vi "Three Button Dialog CORE.vi"(4 "Allow user to close window? (TRUE)":bool=TRUE, 5 "Justify Message (Left)":enum16{"Left", "Center", "Right"}(ring), 6 "Keyboard Shortcuts (Left is <Enter>)":T1={"Left Button Key Shortcut"={"Control"=FALSE, "Shift"=FALSE, "Key"="<Enter>"}, "Center Button Key Shortcut"={"Control"=FALSE, "Shift"=FALSE, "Key"=""}, "Right Button Key Shortcut"={"Control"=FALSE, "Shift"=FALSE, "Key"=""}}, 7 "Window Title (\"\")":string, 8 "Right Button Text (\"Cancel\")":string="Cancel", 9 "Center Button Text (\"No\")":string="No", 10 "Left Button Text (\"Yes\")":string="Yes", 11 "message":string) -> (3 "Which Button?":T2(ring)=enum."Center Button")   [LabVIEW 2020]
doc: "Displays text in a dialog with three buttons. The output enum indicates which of the three buttons the user chose, or it indicates that the user closed the dialog without making any choice."
panel:
  in  "OK":string="OK"
  out "C-Message":string
  in  "Right Button":bool
  in  "Center Button":bool
  in  "Left Button":bool
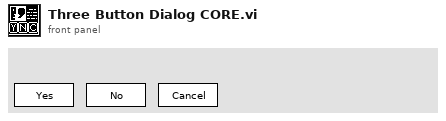
[diagram p1: front panel]
types:
  T1 = cluster{"Left Button Key Shortcut":cluster{"Control":bool, "Shift":bool, "Key":string}, "Center Button Key Shortcut":cluster{"Control":bool, "Shift":bool, "Key":string}, "Right Button Key Shortcut":cluster{"Control":bool, "Shift":bool, "Key":string}}
  T2 = enum16{"Left Button", "Center Button", "Right Button", "Window Close"}
  T3 = cluster{"left":i16, "top":i16, "right":i16, "bottom":i16}
  T4 = cluster{"Control":bool, "Shift":bool, "Key":string}
  T5 = cluster{bool, "Control":bool, "Shift":bool, "Key":string}
  T6 = cluster{"Left":i16, "Top":i16, "Right":i16, "Bottom":i16}
  T7 = typedef "LVRectTypeDef.ctl" = cluster{"Left":i16, "Top":i16, "Right":i16, "Bottom":i16}
  T8 = typedef "LVPointTypeDef.ctl" = cluster{"Horizontal":i16, "Vertical":i16}
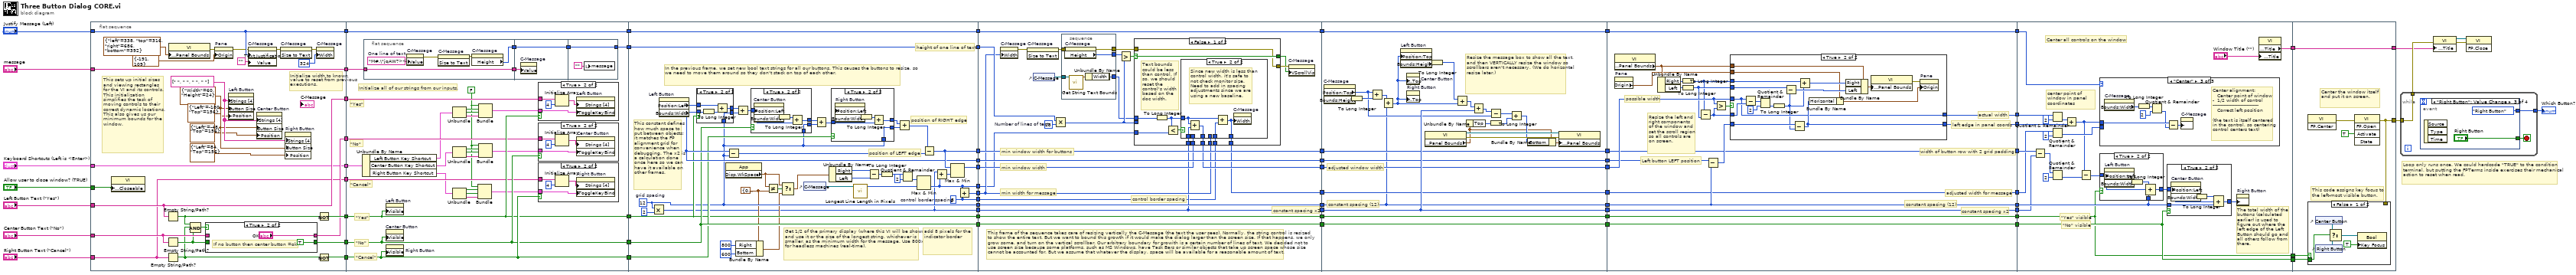
[diagram p0: block diagram]
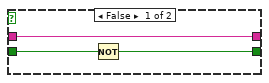
[diagram p2: hidden frame]
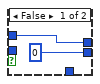
[diagram p6: hidden frame]
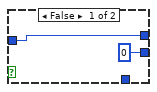
[diagram p7: hidden frame]
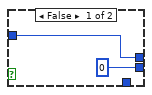
[diagram p8: hidden frame]
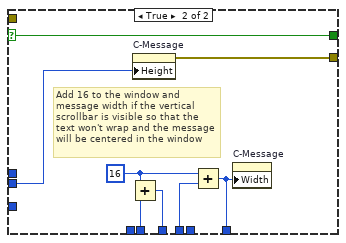
[diagram p10: hidden frame]
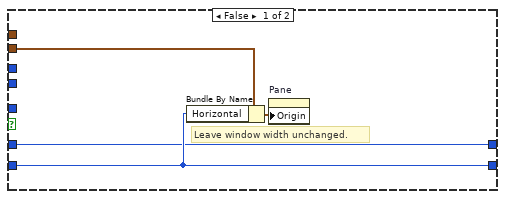
[diagram p11: hidden frame]
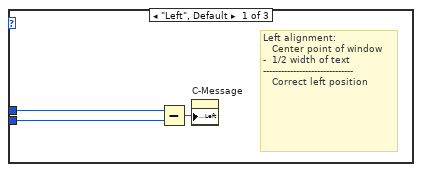
[diagram p12: hidden frame]
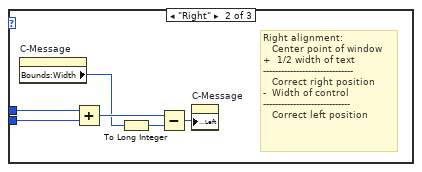
[diagram p13: hidden frame]
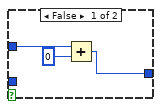
[diagram p14: hidden frame]
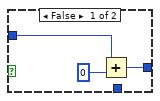
[diagram p15: hidden frame]
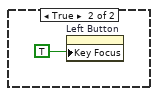
[diagram p16: hidden frame]
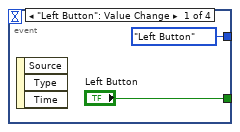
[diagram p17: hidden frame]
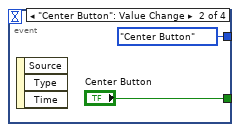
[diagram p18: hidden frame]
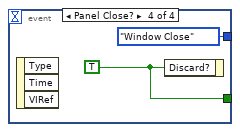
[diagram p19: hidden frame]
diagram:
  # "Loop only runs once. We could hardcode \"TRUE\" to the condition terminal, but putting the FPTerms inside exercises their mechanical action to reset when read."
  n1 = flat-sequence {
    tunnel: [w87] -> w15
    tunnel: [w89] -> w14
    tunnel: [w88] -> w13
    tunnel: [w83] -> w12
    tunnel: [w84] -> w11
    tunnel: [w81] -> w10
    tunnel: [w80] -> w9
    tunnel: "Left Button Text (\"Yes\")" -> [w83]
    tunnel: "Center Button Text (\"No\")" -> [w82]
    tunnel: "Right Button Text (\"Cancel\")" -> [w81]
    tunnel: "Justify Message (Left)" -> [w80]
    tunnel: "Keyboard Shortcuts (Left is <Enter>)" -> [w77]
    tunnel: [w77] -> w8
    tunnel: "message" -> [w76]
    tunnel: [w76] -> w7
    tunnel: "Allow user to close window? (TRUE)" -> [w75]
    tunnel: w15 -> [w131]
    tunnel: [w131] -> w65
    tunnel: w14 -> [w130]
    tunnel: [w130] -> w64
    tunnel: w13 -> [w129]
    tunnel: [w129] -> w63
    tunnel: w12 -> [w128]
    tunnel: w11 -> [w127]
    tunnel: w10 -> [w126]
    tunnel: w9 -> [w125]
    tunnel: [w125] -> w62
    tunnel: [w121] -> w61
    tunnel: w8 -> [w124]
    tunnel: w7 -> [w120]
    tunnel: [w192] -> w60
    tunnel: [w189] -> w59
    tunnel: [w188] -> w58
    tunnel: [w171] -> w57
    tunnel: [w153] -> w56
    tunnel: w65 -> [w181]
    tunnel: w64 -> [w183]
    tunnel: [w183] -> w55
    tunnel: w63 -> [w179]
    tunnel: [w179] -> w54
    tunnel: [w164] -> w53
    tunnel: w62 -> [w174]
    tunnel: [w174] -> w52
    tunnel: w61 -> [w173]
    tunnel: [w173] -> w51
    tunnel: [w162] -> w4
    tunnel: [w161] -> w3
    tunnel: w60 -> [w227]
    tunnel: [w226] -> w50
    tunnel: w59 -> [w233]
    tunnel: [w233] -> w49
    tunnel: w58 -> [w232]
    tunnel: [w232] -> w48
    tunnel: w57 -> [w231]
    tunnel: [w231] -> w47
    tunnel: w56 -> [w220]
    tunnel: [w220] -> w46
    tunnel: w55 -> [w230]
    tunnel: [w230] -> w45
    tunnel: w54 -> [w229]
    tunnel: [w229] -> w44
    tunnel: w53 -> [w221]
    tunnel: [w225] -> w43
    tunnel: w52 -> [w228]
    tunnel: [w228] -> w42
    tunnel: w51 -> [w223]
    tunnel: w4 -> [w219]
    tunnel: w3 -> [w218]
    tunnel: w50 -> [w282]
    tunnel: [w282] -> w41
    tunnel: w49 -> [w281]
    tunnel: [w281] -> w40
    tunnel: w48 -> [w280]
    tunnel: [w280] -> w39
    tunnel: w47 -> [w273]
    tunnel: [w273] -> w38
    tunnel: w46 -> [w290]
    tunnel: [w290] -> w37
    tunnel: w45 -> [w279]
    tunnel: [w279] -> w36
    tunnel: w44 -> [w278]
    tunnel: [w278] -> w35
    tunnel: w43 -> [w277]
    tunnel: [w277] -> w34
    tunnel: w42 -> [w276]
    tunnel: [w276] -> w33
    tunnel: w41 -> [w317]
    tunnel: [w312] -> w32
    tunnel: w40 -> [w305]
    tunnel: [w305] -> w31
    tunnel: w39 -> [w311]
    tunnel: w38 -> [w310]
    tunnel: [w310] -> w30
    tunnel: w37 -> [w304]
    tunnel: [w304] -> w29
    tunnel: [w308] -> w28
    tunnel: w36 -> [w303]
    tunnel: [w303] -> w27
    tunnel: w35 -> [w302]
    tunnel: [w302] -> w26
    tunnel: w34 -> [w299]
    tunnel: [w299] -> w25
    tunnel: w33 -> [w301]
    tunnel: [w301] -> w24
    tunnel: [w342] -> w23
    tunnel: w32 -> [w361]
    tunnel: w31 -> [w354]
    tunnel: w30 -> [w358]
    tunnel: w29 -> [w353]
    tunnel: w28 -> [w360]
    tunnel: w27 -> [w341]
    tunnel: w26 -> [w340]
    tunnel: w25 -> [w346]
    tunnel: w24 -> [w347]
    tunnel: [w341] -> w6
    tunnel: [w340] -> w5
    tunnel: [w396] -> w68
    tunnel: [w398] -> w66
    tunnel: w23 -> [w398]
    tunnel: w6 -> [w394]
    tunnel: w5 -> [w395]
    frame #0 {
      w97 = string[] [" ", " ", " ", " "] ("Strings [4]")
      w96 = cluster{"Width":u32, "Height":u32} {"Width"=60, "Height"=24} ("Button Size")
      # "Initialize width to known value to reset from previous executions."
      # "This sets up initial sizes and viewing rectangles\nfor the VI and its controls. This initialization\nsimplifies the task of moving controls to their\ncorrect dynamic locations. This also gives us our\nminimum bounds for the window."
      n2 = property class="VI"("Front Panel Window:Closeable"=w75) -> ()  [unwired: 2 in, 2 out]
      n3 = Empty String/Path?(string/path=w83) -> (empty?=w91:bool)
      n4 = Empty String/Path?(string/path=w82) -> (empty?=w79:bool)
      n5 = Empty String/Path?(string/path=w81) -> (empty?=w78:bool)
      n6 = property class="VI"("Front Panel Window:Panel Bounds"=T3 {"left"=338, "top"=316, "right"=686, "bottom"=392} ("Front Panel.PanelBounds")) -> (error out=w74:errorcluster)  [unwired: 2 in, 1 out]
      n7 = Compound Arithmetic op=AND(w91, w78, w79) -> (w90:bool)
      n8 = case shown="True" w90 {
        tunnel: w79 -> [w100 _]
        tunnel: [w99 TRUE] -> w89
        tunnel: w82 -> [w98 _]
        tunnel: [w98 "OK"] -> w84
        frame False {
          n9 = Not(x=w100) -> (.not. x?=w99:bool)
        }
        frame True {
          # "If no button then center button =ok"
        }
      }
      n10 = property on="Pane" class="Pane"(error in=w74, "Origin"=cluster{"Horizontal":i16, "Vertical":i16} {"Horizontal"=-191, "Vertical"=109} ("Front Panel.Origin")) -> (error out=w73:errorcluster)  [unwired: 1 in, 1 out]
      n11 = property on="Left Button" class="Bool"("Strings [4]"=w97, "Button Size"=w96, "Position"=cluster{"Left":i32, "Top":i32} {"Left"=-180, "Top"=156}) -> ()  [unwired: 2 in, 2 out]
      n12 = property on="C-Message" class="Str"(error in=w73, "Text.Justification"=w80, "Value"="") -> (error out=w92:errorcluster)  [unwired: 1 in, 1 out]
      n13 = property on="Center Button" class="Bool"("Strings [4]"=w97, "Button Size"=w96, "Position"=cluster{"Left":i32, "Top":i32} {"Left"=-48, "Top"=156}) -> ()  [unwired: 2 in, 2 out]
      n14 = invoke on="C-Message" class="Str" method="Size to Text"(error in=w92) -> (error out=w71:errorcluster)  [unwired: 2 in, 2 out]
      n15 = property on="Right Button" class="Bool"("Strings [4]"=w97, "Button Size"=w96, "Position"=cluster{"Left":i32, "Top":i32} {"Left"=84, "Top"=156}) -> ()  [unwired: 2 in, 2 out]
      n16 = property on="C-Message" class="Str"(error in=w71, "Width"=u32 324 ("Size:Width")) -> ()  [unwired: 1 in, 2 out]
      n17 = Not(x=w91) -> (.not. x?=w88:bool)
      n18 = Not(x=w78) -> (.not. x?=w87:bool)
    }
    frame #1 {
      w105 = FALSE
      # "\"Cancel\""
      # "\"No\""
      # "\"Yes\""
      # "\"Cancel\""
      # "\"No\""
      # "\"Yes\""
      # "Initialize all of our strings from our inputs."
      n19 = Unbundle By Name(w124) -> ("Left Button Key Shortcut"=w118:T4, "Center Button Key Shortcut"=w110:T4, "Right Button Key Shortcut"=w104:T4)
      n20 = flat-sequence {
        tunnel: [w133] -> w123
        tunnel: w120 -> [w132]
        tunnel: [w132] -> w119
        tunnel: w123 -> [w138]
        tunnel: [w138] -> w122
        tunnel: w119 -> [w137]
        tunnel: w122 -> [w139]
        tunnel: [w139] -> w121
        frame #0 {
          w136 = "M#,\"jqAW?><"  # One line of text
          n21 = property on="C-Message" class="Str"("Value"=w136) -> (error out=w134:errorcluster)  [unwired: 2 in, 1 out]
          n22 = invoke on="C-Message" class="Str" method="Size to Text"(error in=w134) -> (error out=w135:errorcluster)  [unwired: 2 in, 2 out]
          n23 = property on="C-Message" class="Str"(error in=w135) -> ("Height"=w133:u32)  [unwired: 1 in, 2 out]
        }
        frame #1 {
          n24 = property on="C-Message" class="Str"("Value"=w137) -> ()  [unwired: 2 in, 2 out]
        }
        frame #2 {
          n25 = local write "message"("") -> ()
        }
      }
      n26 = property on="Left Button" class="Bool"("Visible"=w129) -> ()  [unwired: 2 in, 2 out]
      n27 = property on="Center Button" class="Bool"("Visible"=w130) -> ()  [unwired: 2 in, 2 out]
      n28 = property on="Right Button" class="Bool"("Visible"=w131) -> ()  [unwired: 2 in, 2 out]
      n29 = Unbundle(w118) -> ("Control"=w117:bool, "Shift"=w116:bool, "Key"=w115:string)
      n30 = Unbundle(w110) -> ("Control"=w113:bool, "Shift"=w112:bool, "Key"=w111:string)
      n31 = Unbundle(w104) -> ("Control"=w108:bool, "Shift"=w107:bool, "Key"=w106:string)
      n32 = Bundle(w105, "Control"=w108, "Shift"=w107, "Key"=w106) -> (w103:T5)  [unwired: 1 in]
      n33 = Bundle(w105, "Control"=w117, "Shift"=w116, "Key"=w115) -> (w114:T5)  [unwired: 1 in]
      n34 = Bundle(w105, "Control"=w113, "Shift"=w112, "Key"=w111) -> (w109:T5)  [unwired: 1 in]
      n35 = case shown="True" w129 {
        tunnel: w128 -> [_ w150]
        tunnel: w114 -> [_ w149]
        frame False {
        }
        frame True {
          n36 = Initialize Array(w150, 4 ("dimension size")) -> (w152:string[])
          n37 = property on="Left Button" class="Bool"("Strings [4]"=w152, "ToggleKeyBind"=w149) -> ()  [unwired: 2 in, 2 out]
        }
      }
      n38 = case shown="True" w130 {
        tunnel: w109 -> [_ w146]
        tunnel: w127 -> [_ w145]
        frame False {
        }
        frame True {
          n39 = Initialize Array(w145, 4 ("dimension size")) -> (w148:string[])
          n40 = property on="Center Button" class="Bool"("Strings [4]"=w148, "ToggleKeyBind"=w146) -> ()  [unwired: 2 in, 2 out]
        }
      }
      n41 = case shown="True" w131 {
        tunnel: w103 -> [_ w142]
        tunnel: w126 -> [_ w141]
        frame False {
        }
        frame True {
          n42 = Initialize Array(w141, 4 ("dimension size")) -> (w144:string[])
          n43 = property on="Right Button" class="Bool"("Strings [4]"=w144, "ToggleKeyBind"=w142) -> ()  [unwired: 2 in, 2 out]
        }
      }
    }
    frame #2 {
      w158 = T6 {"Left"=0, "Top"=0, "Right"=0, "Bottom"=0} ("Display:Primary Workspace")
      w162 = 8  # control border spacing
      w171 = 12  # grid spacing
      # "position of RIGHT edge"
      # "height of one line of text"
      # "add 8 pixels for the indicator border"
      # "Get 1/2 of the primary display (where this VI will be shown) and use it or the size of the longest string, whichever is smaller, as the minimum width for the message. Use 800x600 for headless machines (real-time)."
      # "This constant defines how much space to put between objects; it matches the FP alignment grid for convenience when debugging. The x2 is a calculation done once here so we can have it available on other frames."
      # "In the previous frame, we set new bool text strings for all our buttons. This causes the buttons to resize, so we need to move them around so they don't stack on top of each other."
      # "position of LEFT edge"
      n44 = Multiply(x=w171, y=2) -> (x*y=w153:i32)
      n45 = property on="Left Button" class="Bool"() -> ("Position:Left"=w188:i32, "Bounds:Width"=w185:u32)  [unwired: 2 in, 2 out]
      n46 = case shown="True" w179 {
        tunnel: w188 -> [w195 w200]
        tunnel: w185 -> [_ w199]
        tunnel: [w195 w198] -> w180
        tunnel: w171 -> [_ w196]
        tunnel: [0 w196] -> w178
        frame False {
        }
        frame True {
          n47 = To Long Integer(number=w199) -> (32bit integer=w197:i32)
          n48 = Add(x=w200, y=w197) -> (x+y=w198:i32)
        }
      }
      n49 = property class="App"() -> ("Disp.WkSpace"=w159:T7)  [unwired: 2 in, 2 out]
      n50 = Subtract(x=w188, y=w171) -> (x-y=w190:i32)
      n51 = Bundle By Name(cluster=w158, "Right"=i16 800, "Bottom"=i16 600) -> (w155:T6)
      n52 = Add(x=w180, y=w178) -> (x+y=w186:i32)
      n53 = case shown="True" w183 {
        tunnel: w186 -> [w209 w214]
        tunnel: [w209 w213] -> w184
        tunnel: [0 w210] -> w177
        tunnel: w171 -> [_ w210]
        frame False {
        }
        frame True {
          n54 = property on="Center Button" class="Bool"("Position:Left"=w214) -> ("Bounds:Width"=w212:u32)  [unwired: 2 in, 2 out]
          n55 = To Long Integer(number=w212) -> (32bit integer=w211:i32)
          n56 = Add(x=w211, y=w214) -> (x+y=w213:i32)
        }
      }
      n57 = Not Equal?(x=w159, y=w158) -> (x != y?=w160:bool)
      n58 = Select(t=w159, s=w160, f=w155) -> (s? t:f=w154:T7)
      n59 = control-ref of="C-Message"() -> (w175:refnum<vi>)
      n60 = Add(x=w184, y=w177) -> (x+y=w187:i32)
      n61 = Unbundle By Name(w154) -> ("Right"=w167:i16, "Left"=w166:i16)
      n62 = case shown="True" w181 {
        tunnel: w187 -> [w202 w207]
        tunnel: [w202 w203] -> w182
        tunnel: [0 w204] -> w176
        tunnel: w171 -> [_ w204]
        frame False {
        }
        frame True {
          n63 = property on="Right Button" class="Bool"("Position:Left"=w207) -> ("Bounds:Width"=w206:u32)  [unwired: 2 in, 2 out]
          n64 = To Long Integer(number=w206) -> (32bit integer=w205:i32)
          n65 = Add(x=w205, y=w207) -> (x+y=w203:i32)
        }
      }
      n66 = call "Longest Line Length in Pixels.vi"("String"=w175) -> ("longest line length"=w168:i32)  [unwired: 9 in]
      n67 = Subtract(x=w167, y=w166) -> (x-y=w170:i16)
      n68 = To Long Integer(number=w170) -> (32bit integer=w165:i32)
      n69 = Add(x=w182, y=w176) -> (x+y=w191:i32)
      n70 = Quotient & Remainder(x=w165, y=2) -> (floor(x/y)=w163:i32)  [unwired: 1 out]
      n71 = Max & Min(x=w163, y=w168) -> (min(x,y)=w161:i32)  [unwired: 1 out]
      n72 = Subtract(x=w191, y=w190) -> (x-y=w189:i32)
      n73 = Add(x=w153, y=w161) -> (x+y=w193:i32)
      n74 = Max & Min(x=w189, y=w193) -> (max(x,y)=w192:i32)  [unwired: 1 out]
      n75 = Add(x=w161, y=w162) -> (x+y=w164:i32)
    }
    frame #3 {
      w235 = u32 25  # Number of lines of text
      # "control border spacing"
      # "constant spacing x2"
      # "min window width for buttons"
      # "min window width"
      # "min width for message"
      # "This frame of the sequence takes care of resizing vertically the C-Message (the text the user sees). Normally, the string control is resized to show the entire text. But we want to bound this growth if it would make the dialog larger than the screen size. If that happens, we only grow some, and turn on the vertical scrollbar. Our arbitrary boundary for growith is a certain number of lines of text. We decided not to use screen size because some platforms, such as MS Windows, have Task Bars or similar objects that take up screen space whose size cannot be accounted for. But we assume that whatever the display, space will be available for a reasonable amount of text."
      n76 = property on="C-Message" class="Str"("Width"=w221) -> (error out=w224:errorcluster)  [unwired: 2 in, 1 out]
      n77 = invoke on="C-Message" class="Str" method="Size to Text"(error in=w224) -> (error out=w239:errorcluster)  [unwired: 2 in, 2 out]
      n78 = control-ref of="C-Message"() -> (w216:refnum<vi>)
      n79 = Multiply(x=w223, y=w235) -> (x*y=w234:u32)
      n80 = stacked-sequence {
        tunnel: w239 -> [w245]
        tunnel: [w244] -> w222
        tunnel: [w243] -> w217
        tunnel: w216 -> [w242]
        tunnel: [w240] -> w215
        frame #0 {
          n81 = property on="C-Message" class="Str"(error in=w245) -> (error out=w243:errorcluster, "Height"=w244:u32)  [unwired: 1 in, 1 out]
          n82 = call "Get String Text Bounds.vi"("String"=w242) -> ("Text bounds"=w241:cluster{"Width":u32, "Height":u32})  [unwired: 10 in]
          n83 = Unbundle By Name(w241) -> ("Width"=w240:u32)
        }
      }
      n84 = Greater?(x=w222, y=w234) -> (0:w238:bool)
      n85 = case shown="False" w238 {
        selector: w238 -> [w257 w271]
        tunnel: [w256 w272] -> w237
        tunnel: [w257 w271] -> w236
        tunnel: w217 -> [w256 _]
        tunnel: w234 -> [_ w270]
        tunnel: [w250 w268] -> w226
        tunnel: w227 -> [w252 w269]
        tunnel: [w249 w265] -> w225
        tunnel: w221 -> [w251 w267]
        tunnel: w215 -> [w254 _]
        tunnel: w218 -> [w253 _]
        tunnel: w220 -> [w248 _]
        tunnel: w219 -> [w247 _]
        frame False {
          # "Text bounds could be less than control. If so, we should reset the control's width based on the doc width."
          n86 = To Long Integer(number=w254) -> (32bit integer=w246:i32)
          n87 = Less?(x=w246, y=w253) -> (x < y?=w255:bool)
          n88 = case shown="True" w255 {
            tunnel: w246 -> [_ w263]
            tunnel: w252 -> [w259 _]
            tunnel: w251 -> [w258 _]
            tunnel: [w259 w262] -> w250
            tunnel: [w258 w261] -> w249
            tunnel: w248 -> [_ w264]
            tunnel: w247 -> [_ w260]
            frame False {
            }
            frame True {
              # "Since new width is less than control width, it's safe to not check monitor size. \nNeed to add in spacing adjustments since we are using a new baseline."
              n89 = Add(x=w263, y=w264) -> (x+y=w262:i32)
              n90 = Add(x=w263, y=w260) -> (x+y=w261:i32)
              n91 = property on="C-Message" class="Str"("Width"=w261) -> ()  [unwired: 2 in, 2 out]
            }
          }
        }
        frame True {
          w266 = 16 ("x")
          # "Add 16 to the window and message width if the vertical scrollbar is visible so that the text won't wrap and the message will be centered in the window"
          n92 = Add(x=w266, y=w269) -> (x+y=w268:i32)
          n93 = property on="C-Message" class="Str"("Height"=w270) -> (error out=w272:errorcluster)  [unwired: 2 in, 1 out]
          n94 = Add(x=w266, y=w267) -> (x+y=w265:i32)
          n95 = property on="C-Message" class="Str"("Width"=w265) -> ()  [unwired: 2 in, 2 out]
        }
      }
      n96 = property on="C-Message" class="Str"(error in=w237, "VScrollVis"=w236) -> ()  [unwired: 1 in, 2 out]
    }
    frame #4 {
      # "adjusted window width"
      # "constant spacing (12)"
      # "Resize the message box to show all the text, and then VERTICALLY resize the window so scrollbars aren't necessary. (We do horizontal resize later.)"
      n97 = property on="C-Message" class="Str"() -> ("Position:Top"=w284:i32, "Bounds:Height"=w283:u32)  [unwired: 2 in, 2 out]
      n98 = To Long Integer(number=w283) -> (32bit integer=w289:i32)
      n99 = Add(x=w284, y=w289) -> (x+y=w274:i32)
      n100 = Add(x=w274, y=w273) -> (x+y=w275:i32)
      n101 = property on="Left Button" class="Bool"("Position:Top"=w275) -> ("Bounds:Height"=w286:u32)  [unwired: 2 in, 2 out]
      n102 = property on="Center Button" class="Bool"("Position:Top"=w275) -> ()  [unwired: 2 in, 2 out]
      n103 = property on="Right Button" class="Bool"("Position:Top"=w275) -> ()  [unwired: 2 in, 2 out]
      n104 = property class="VI"() -> (reference out=w296:refnum<vi>, error out=w297:errorcluster, "Front Panel Window:Panel Bounds"=w287:T7)  [unwired: 2 in]
      n105 = To Long Integer(number=w286) -> (32bit integer=w285:i32)
      n106 = Add(x=w285, y=w275) -> (x+y=w291:i32)
      n107 = Unbundle By Name(w287) -> ("Top"=w294:i16)
      n108 = Add(x=w291, y=w290) -> (x+y=w292:i32)
      n109 = Subtract(x=w292, y=w284) -> (x-y=w295:i32)
      n110 = To Long Integer(number=w294) -> (32bit integer=w288:i32)
      n111 = Add(x=w295, y=w288) -> (x+y=w293:i32)
      n112 = Bundle By Name(cluster=w287, "Bottom"=w293) -> (w298:T7)
      n113 = property class="VI"(reference=w296, error in=w297, "Front Panel Window:Panel Bounds"=w298) -> ()  [unwired: 2 out]
    }
    frame #5 {
      # "adjusted width for message"
      # "constant spacing x2"
      # "constant spacing (12)"
      # "Left button LEFT position"
      # "left edge in panel coords"
      # "width of button row with 2 grid padding"
      # "Resize the left and\nright components\nof the window and\nset the scroll region\nso all controls are \non screen."
      # "actual width"
      # "possible width"
      n114 = property class="VI"() -> ("Front Panel Window:Panel Bounds"=w314:T7)  [unwired: 2 in, 2 out]
      n115 = property on="Pane" class="Pane"() -> ("Origin"=w300:T8)  [unwired: 2 in, 2 out]
      n116 = Unbundle By Name(w314) -> ("Right"=w316:i16, "Left"=w315:i16)
      n117 = To Long Integer(number=w316) -> (32bit integer=w306:i32)
      n118 = To Long Integer(number=w315) -> (32bit integer=w307:i32)
      n119 = Subtract(x=w306, y=w307) -> (x-y=w318:i32)
      n120 = Subtract(x=w311, y=w310) -> (x-y=w309:i32)
      n121 = Greater?(x=w317, y=w318) -> (0:w313:bool)
      n122 = case shown="True" w313 {
        tunnel: w318 -> [w320 w339]
        tunnel: w317 -> [_ w326]
        tunnel: w306 -> [_ w334]
        tunnel: w307 -> [_ w335]
        tunnel: w314 -> [_ w336]
        tunnel: [w322 w328] -> w312
        tunnel: w300 -> [w321 w329]
        tunnel: w309 -> [w322 w327]
        tunnel: [w320 w326] -> w308
        frame False {
          # "Leave window width unchanged."
          n123 = Bundle By Name(cluster=w321, "Horizontal"=w322) -> (w319:T8)
          n124 = property on="Pane" class="Pane"("Origin"=w319) -> ()  [unwired: 2 in, 2 out]
        }
        frame True {
          n125 = Subtract(x=w326, y=w339) -> (x-y=w338:i32)
          n126 = Quotient & Remainder(x=w338, y=2) -> (floor(x/y)=w331:i32)  [unwired: 1 out]
          n127 = To Long Integer(number=w331) -> (32bit integer=w325:i32)
          n128 = Subtract(x=w335, y=w325) -> (x-y=w332:i32)
          n129 = Subtract(x=w327, y=w325) -> (x-y=w328:i32)
          n130 = Add(x=w334, y=w325) -> (x+y=w333:i32)
          n131 = Bundle By Name(cluster=w329, "Horizontal"=w328) -> (w323:T8)
          n132 = Bundle By Name(cluster=w336, "Right"=w333, "Left"=w332) -> (w330:T7)
          n133 = property class="VI"("Front Panel Window:Panel Bounds"=w330) -> (error out=w324:errorcluster)  [unwired: 2 in, 1 out]
          n134 = property on="Pane" class="Pane"(error in=w324, "Origin"=w323) -> ()  [unwired: 1 in, 2 out]
        }
      }
    }
    frame #6 {
      # "\"No\" visible"
      # "\"Yes\" visible"
      # "The total width of the buttons (calculated earlier) is used to figure out where the left edge of the Left Button should go and all others follow from there."
      # "center point of window in panel coordinates"
      # "Center all controls on the window"
      n135 = Subtract(x=w354, y=w353) -> (x-y=w355:i32)
      n136 = Quotient & Remainder(x=w360, y=2) -> (floor(x/y)=w357:i32)  [unwired: 1 out]
      n137 = Quotient & Remainder(x=w346, y=2) -> (floor(x/y)=w345:i32)  [unwired: 1 out]
      n138 = Quotient & Remainder(x=w355, y=2) -> (floor(x/y)=w352:i32)  [unwired: 1 out]
      n139 = Add(x=w357, y=w361) -> (x+y=w344:i32)
      n140 = Subtract(x=w344, y=w352) -> (x-y=w351:i32)
      n141 = case shown="\"Center\"" w347 {
        tunnel: w344 -> [w364 w370 w372]
        tunnel: w345 -> [w362 w369 _]
        frame "Left", Default {
          # "Left alignment:\n   Center point of window\n-  1/2 width of text\n------------------------------\n   Correct left position"
          n142 = Subtract(x=w364, y=w362) -> (x-y=w363:i32)
          n143 = property on="C-Message" class="Str"("Position:Left"=w363) -> ()  [unwired: 2 in, 2 out]
        }
        frame "Right" {
          # "Right alignment:\n   Center point of window\n+  1/2 width of text\n------------------------------\n   Correct right position\n-  Width of control\n-----------------------------\n   Correct left position"
          n144 = property on="C-Message" class="Str"() -> ("Bounds:Width"=w366:u32)  [unwired: 2 in, 2 out]
          n145 = Add(x=w370, y=w369) -> (x+y=w368:i32)
          n146 = To Long Integer(number=w366) -> (32bit integer=w365:i32)
          n147 = Subtract(x=w368, y=w365) -> (x-y=w367:i32)
          n148 = property on="C-Message" class="Str"("Position:Left"=w367) -> ()  [unwired: 2 in, 2 out]
        }
        frame "Center" {
          # "Center alignment:\n   Center point of window\n-  1/2 width of control\n------------------------------\n   Correct left position\n\n(the text is itself centered in the control, so centering control centers text)"
          n149 = property on="C-Message" class="Str"() -> ("Bounds:Width"=w375:u32)  [unwired: 2 in, 2 out]
          n150 = To Long Integer(number=w375) -> (32bit integer=w373:i32)
          n151 = Quotient & Remainder(x=w373, y=2) -> (floor(x/y)=w371:i32)  [unwired: 1 out]
          n152 = Subtract(x=w372, y=w371) -> (x-y=w374:i32)
          n153 = property on="C-Message" class="Str"("Position:Left"=w374) -> ()  [unwired: 2 in, 2 out]
        }
      }
      n154 = case shown="True" w340 {
        tunnel: w358 -> [_ w392]
        tunnel: w351 -> [w387 w391]
        tunnel: [w386 w389] -> w350
        frame False {
          n155 = Add(x=w387, y=0) -> (x+y=w386:i32)
        }
        frame True {
          n156 = property on="Left Button" class="Bool"("Position:Left"=w391) -> ("Bounds:Width"=w390:u32)  [unwired: 2 in, 2 out]
          n157 = To Long Integer(number=w390) -> (32bit integer=w388:i32)
          n158 = Compound Arithmetic op=ADD(w388, w391, w392) -> (w389:i32)
        }
      }
      n159 = case shown="True" w341 {
        tunnel: w358 -> [_ w384]
        tunnel: w350 -> [w379 w382]
        tunnel: [w378 w381] -> w349
        frame False {
          n160 = Add(x=w379, y=0) -> (x+y=w378:i32)
        }
        frame True {
          n161 = property on="Center Button" class="Bool"("Position:Left"=w382) -> ("Bounds:Width"=w383:u32)  [unwired: 2 in, 2 out]
          n162 = To Long Integer(number=w383) -> (32bit integer=w380:i32)
          n163 = Compound Arithmetic op=ADD(w380, w382, w384) -> (w381:i32)
        }
      }
      n164 = property on="Right Button" class="Bool"("Position:Left"=w349) -> ()  [unwired: 2 in, 2 out]
      n165 = property class="VI"("Front Panel Window:Title"="Window Title (\"\")") -> ("Front Panel Window:Title"=w342:string)  [unwired: 2 in, 2 out]
    }
    frame #7 {
      # "This code assigns key focus to\nthe left-most visible button."
      # "Center the window itself and put it on screen."
      n166 = invoke class="VI" method="FP.Center"() -> (error out=w397:errorcluster)  [unwired: 3 in, 2 out]
      n167 = invoke class="VI" method="FP.Open"(error in=w397, "Activate"=TRUE ("Front Panel Window:Open")) -> (error out=w396:errorcluster)  [unwired: 3 in, 4 out]
      n168 = case shown="False" w395 {
        tunnel: w396 -> [_ _]
        tunnel: w394 -> [w403 _]
        frame False {
          n169 = control-ref of="Center Button"() -> (w402:refnum<vi>)
          n170 = control-ref of="Right Button"() -> (w401:refnum<vi>)
          n171 = Select(t=w402, s=w403, f=w401) -> (s? t:f=w400:refnum<vi>)
          n172 = property class="Bool"(reference=w400, "Key Focus"=TRUE) -> ()  [unwired: 1 in, 2 out]
        }
        frame True {
          n173 = property on="Left Button" class="Bool"("Key Focus"=TRUE) -> ()  [unwired: 2 in, 2 out]
        }
      }
    }
  }
  n174 = while {
    tunnel: [w407] -> w69
    tunnel: [w406] -> w67
    tunnel: w68 -> [w406]
    stop <- w405 stop-if-true
    n175 = event shown="[2] \"Right Button\": Value Change" {
      selector: _ -> [_ _ _ _]
      dyn-events: _ -> [_ _ _ _]
      timeout: _ -> [_ _ _ _]
      tunnel: ["Left Button" "Center Button" "Right Button" w414] -> w405
      tunnel: [T2."Left Button" ("Which Button?") T2."Center Button" ("Which Button?") T2."Right Button" ("Which Button?") T2."Window Close" ("Which Button?")] -> w407
      event "Left Button": Value Change {
        n176 = event-data() -> ()  [unwired: 1 in, 3 out]
      }
      event "Center Button": Value Change {
        n177 = event-data() -> ()  [unwired: 1 in, 3 out]
      }
      event "Right Button": Value Change {
        n178 = event-data() -> ()  [unwired: 1 in, 3 out]
      }
      event Panel Close? {
        w414 = TRUE ("Discard?")
        n179 = event-data() -> ()  [unwired: 1 in, 3 out]
        n180 = event-data("Discard?"=w414) -> ()  [unwired: 1 in, 1 out]
      }
    }
  }
  "Which Button?" <- w69
  n181 = property class="VI"(error in=w67, "Front Panel Window:Title"=w66) -> (reference out=w1:refnum<vi>, error out=w2:errorcluster)  [unwired: 1 in]
  n182 = invoke class="VI" method="FP.Close"(reference=w1, error in=w2) -> ()  [unwired: 1 in, 3 out]
